vi "CleanUp.vi"(0 "object in":refnum<class "TDMSlogg.lvclass">, 5 "error in (no error)":errorcluster) -> (14 "object out":refnum<class "TDMSlogg.lvclass">, 19 "error out":errorcluster)   [LabVIEW 2019, in "TDMSlogg.lvclass"]
uses:
  TDMSlogg.lvclass
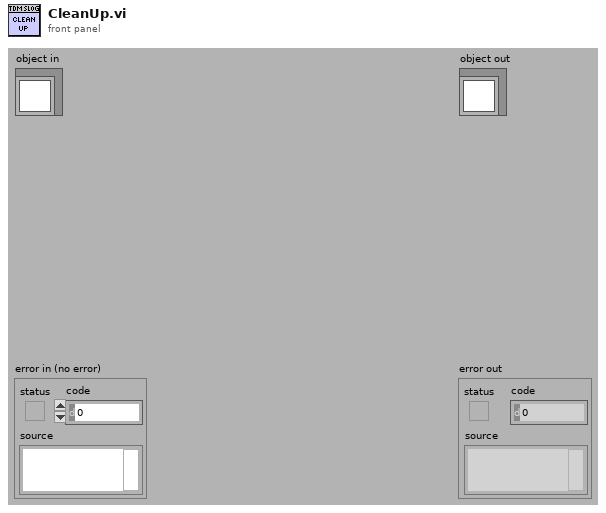
[diagram p1: front panel]
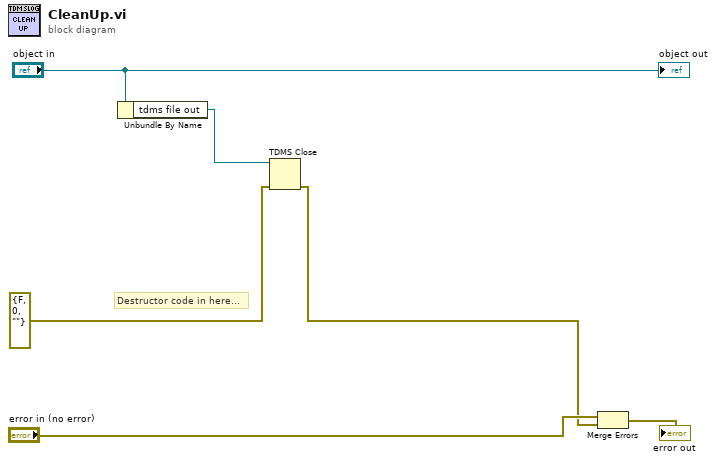
[diagram p0: block diagram]
diagram:
  # "Destructor code in here..."
  n1 = Unbundle By Name("object in") -> ("tdms file out"=w3:refnum<k34>)
  n2 = TDMS Close(8:errorcluster {"status"=FALSE, "code"=0, "source"=""} ("error in (no error)"), 11:w3) -> (0:w1:errorcluster)  [unwired: 1 out]
  n3 = Merge Errors("error in (no error)", w1) -> (→"error out":errorcluster)
  "object out" <- "object in"
